vi "RSZVB Set IMOD Internal Combiner.vi"(8 "error in (no error)":errorcluster {"code" format="%.0x"}, 9 "Internal Combiner (T: On)":bool=TRUE, 10 "Channel (1)":i32=1, 11 "VISA session":refnum<visa-resource-name>) -> (0 "error out":errorcluster {"code" format="%.0x"}, 3 "dup VISA session":refnum<visa-resource-name>)   [LabVIEW 2011]
doc: "This VI enables or disables the internal combiner. The internal combiner requires the following port configuration: Lower Tone: Port 1, Upper Tone: Port 3.\n\nNote(s):\n\n(1) This VI requires option R&S ZVT20-B11.\n\nRemote-control command(s):\n[SENSe<Ch>:]FREQuency:IMODulation:COMBiner[:STATe] ON | OFF"
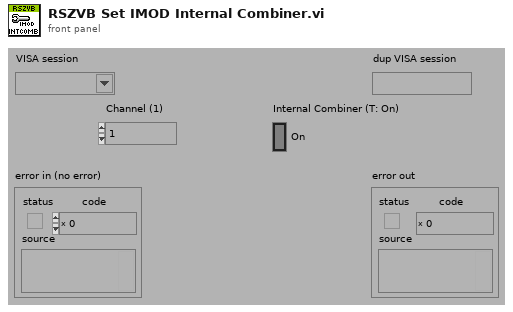
[diagram p1: front panel]
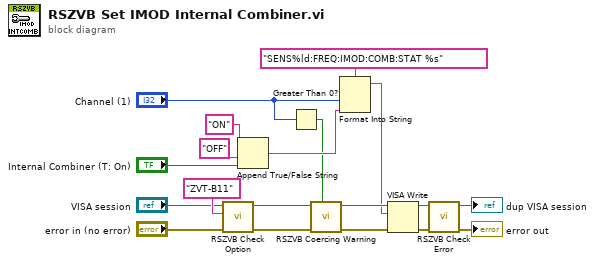
[diagram p0: block diagram]
diagram:
  n1 = call "RSZVB Check Option.vi"("error in (no error)"="error in (no error)", "Options"="ZVT-B11", "VISA session"="VISA session") -> ("error out"=w5:errorcluster, "dup VISA session"=w6:refnum<visa-resource-name>)  [unwired: 7 in]
  n2 = Append True/False String(1:"Internal Combiner (T: On)", 2:"OFF" ("false string"), 3:"ON" ("true string")) -> (0:w12:string)  [unwired: 1 in]
  n3 = Greater Than 0?(x="Channel (1)") -> (x > 0?=w4:bool)
  n4 = call "RSZVB Coercing Warning.vi"("In Range?"=w4, "error in (no error)"=w5, "VISA session"=w6) -> ("error out"=w9:errorcluster, "dup VISA session"=w10:refnum<visa-resource-name>)  [unwired: 7 in]
  n5 = Format Into String(format string="SENS%ld:FREQ:IMOD:COMB:STAT %s", "Channel (1)", w12) -> (resulting string=w3:string)  [unwired: 2 in, 1 out]
  n6 = VISA Write(VISA resource name=w10, write buffer=w3, error in (no error)=w9) -> (VISA resource name out=w8:refnum<visa-resource-name>, error out=w7:errorcluster)  [unwired: 1 out]
  n7 = call "RSZVB Check Error.vi"("error in (no error)"=w7, "VISA session"=w8) -> ("error out"=→"error out":errorcluster, "dup VISA session"=→"dup VISA session":refnum<visa-resource-name>)  [unwired: 8 in]
